vi "Collect IO Control Names.vi"(0 "IO Control":refnum<vi>, 5 "IO Controls in":string[](array[string]), 7 "DAQ Controls in":string[](array[string]), 11 "error in (no error)":errorcluster) -> (4 "IO Controls out":string[](array[string]), 6 "DAQ Controls out":string[](array[string]), 15 "error out":errorcluster)   [LabVIEW 2021, in "Migrator.lvlib"]
uses:
  Migrator.lvlib
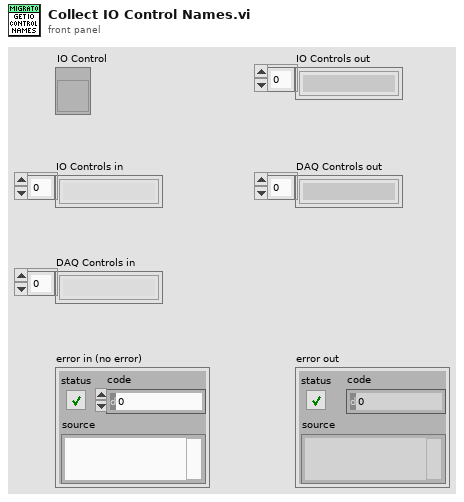
[diagram p1: front panel]
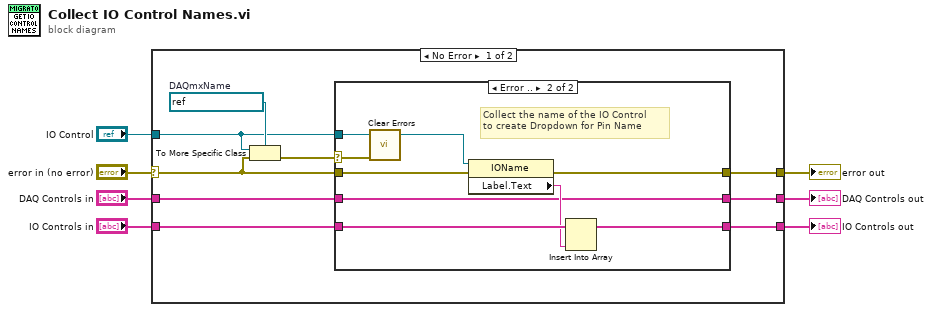
[diagram p0: block diagram]
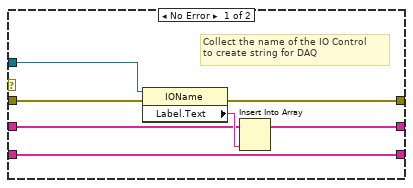
[diagram p2: hidden frame]
diagram:
  n1 = case shown="No Error" "error in (no error)" {
    selector: "error in (no error)" -> [w8 w34]
    tunnel: [w16 w33] -> w7
    tunnel: "DAQ Controls in" -> [w15 w33]
    tunnel: "IO Control" -> [w13 _]
    tunnel: [w12 w32] -> w3
    tunnel: "IO Controls in" -> [w11 w32]
    tunnel: [w10 w34] -> w1
    frame No Error {
      w14 = refnum<vi> refnum  # DAQmxName
      n2 = To More Specific Class(target class=w14, reference=w13, error in=w8) -> (error out=w9:errorcluster)  [unwired: 1 out]
      n3 = case shown="Error .." w9 {
        selector: w9 -> [_ w24]
        tunnel: [w18 w31] -> w10
        tunnel: w11 -> [w23 w30]
        tunnel: [w23 w28] -> w12
        tunnel: w13 -> [w17 w26]
        tunnel: w15 -> [w21 w25]
        tunnel: [w20 w25] -> w16
        tunnel: w8 -> [w19 w27]
        frame No Error {
          # "Collect the name of the IO Control \nto create string for DAQ"
          n4 = property class="IOName"(reference=w17, error in=w19) -> (error out=w18:errorcluster, "Label.Text"=w22:string)  [unwired: 1 out]
          n5 = Insert Into Array(array=w21, new element=w22) -> (w20:string[])  [unwired: 1 in]
        }
        frame Error {
          # "Collect the name of the IO Control \nto create Dropdown for Pin Name"
          n6 = call <vilib>:"Clear Errors.vi"("error in (no error)"=w24) -> ()  [unwired: 5 in, 2 out]
          n7 = property class="IOName"(reference=w26, error in=w27) -> (error out=w31:errorcluster, "Label.Text"=w29:string)  [unwired: 1 out]
          n8 = Insert Into Array(array=w30, new element=w29) -> (w28:string[])  [unwired: 1 in]
        }
      }
    }
    frame Error {
    }
  }
  "DAQ Controls out" <- w7
  "IO Controls out" <- w3
  "error out" <- w1
